vi "TCP-Send Error.vi"(0 "connection ID":refnum<k5>, 11 "error in (no error)":errorcluster) -> (15 "error out":errorcluster)   [LabVIEW 2020]
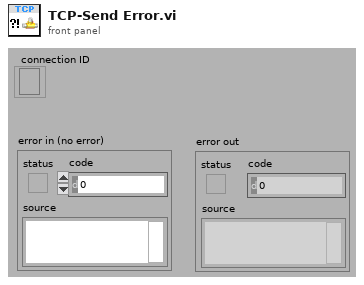
[diagram p1: front panel]
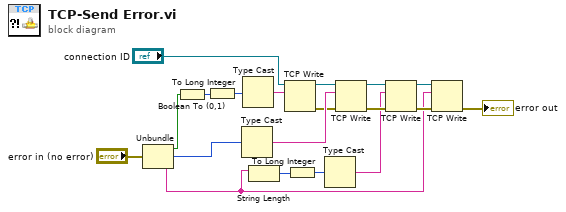
[diagram p0: block diagram]
diagram:
  n1 = Unbundle("error in (no error)") -> ("status"=w18:bool, "code"=w15:i32, "source"=w7:string)
  n2 = Boolean To (0,1)(Boolean=w18) -> (0, 1=w17:i16)
  n3 = To Long Integer(number=w17) -> (32bit integer=w16:i32)
  n4 = Type Cast(x=w15) -> (*(type *) &x=w14:string)  [unwired: 1 in]
  n5 = Type Cast(x=w16) -> (*(type *) &x=w19:string)  [unwired: 1 in]
  n6 = String Length(string=w7) -> (length=w6:i32)
  n7 = TCP Write(connection ID="connection ID", data in=w19) -> (connection ID out=w12:refnum<k5>, error out=w13:errorcluster)  [unwired: 2 in, 1 out]
  n8 = To Long Integer(number=w6) -> (32bit integer=w5:i32)
  n9 = Type Cast(x=w5) -> (*(type *) &x=w4:string)  [unwired: 1 in]
  n10 = TCP Write(connection ID=w12, data in=w14, error in (no error)=w13) -> (connection ID out=w11:refnum<k5>, error out=w9:errorcluster)  [unwired: 1 in, 1 out]
  n11 = TCP Write(connection ID=w11, data in=w4, error in (no error)=w9) -> (connection ID out=w10:refnum<k5>, error out=w8:errorcluster)  [unwired: 1 in, 1 out]
  n12 = TCP Write(connection ID=w10, data in=w7, error in (no error)=w8) -> (error out=→"error out":errorcluster)  [unwired: 1 in, 2 out]
